vi "myRIO_BRig_RT_dataExp_TPB_max__R.vi"() -> (2 "output_TPB_max__R":i32)   [LabVIEW 2014]
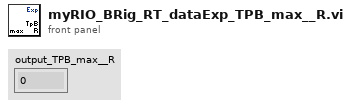
[diagram p1: front panel]
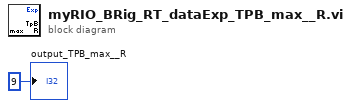
[diagram p0: block diagram]
diagram:
  "output_TPB_max__R" <- 9 ("output_iBlock")
